vi "VISA Factory.vi"(8 "error in (no error)":errorcluster, 10 "VISA settings":T1) -> (0 "error out":errorcluster, 3 "protocol out":refnum<class "Protocol Parent.lvclass">)   [LabVIEW 2023, in "Protocols.lvlib" / "VISA.lvclass"]
doc: "Instantiates a new VISA Protocol object using the provided VISA settings."
uses:
  VISA.lvclass
  Protocol Parent/Protocol Parent.lvclass
  VISA Settings.ctl
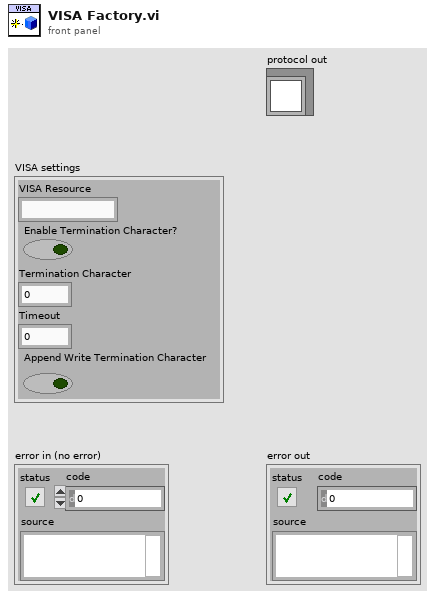
[diagram p1: front panel]
types:
  T1 = typedef "Protocols.lvlib/VISA.lvclass/VISA Settings.ctl" = cluster{"VISA Resource":string, "Enable Termination Character?":bool, "Termination Character":u8, "Timeout":u32, "Append Write Termination Character":bool}
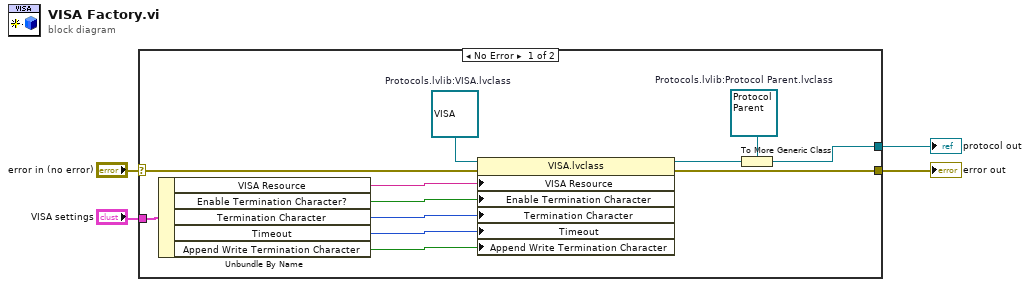
[diagram p0: block diagram]
diagram:
  n1 = case shown="No Error" "error in (no error)" {
    selector: "error in (no error)" -> [w8 w17]
    tunnel: "VISA settings" -> [w16 _]
    tunnel: [w5 _] -> w1
    tunnel: [w9 w17] -> w3
    frame No Error {
      w6 = refnum<class "Protocol Parent.lvclass"> refnum  # Protocols.lvlib:Protocol Parent.lvclass
      w15 = refnum<class "VISA.lvclass"> refnum  # Protocols.lvlib:VISA.lvclass
      n2 = Unbundle By Name(w16) -> ("VISA Resource"=w14:string, "Enable Termination Character?"=w13:bool, "Termination Character"=w12:u8, "Timeout"=w11:u32, "Append Write Termination Character"=w10:bool)
      n3 = property class="VISA.lvclass"(reference=w15, error in=w8, "VISA Resource"=w14, "Enable Termination Character"=w13, "Termination Character"=w12, "Timeout"=w11, "Append Write Termination Character"=w10) -> (reference out=w7:refnum<class "VISA.lvclass">, error out=w9:errorcluster)
      n4 = To More Generic Class(target class=w6, reference=w7) -> (generic class reference=w5:refnum<class "Protocol Parent.lvclass">)
    }
    frame Error {
    }
  }
  "error out" <- w3
  "protocol out" <- w1
